vi "Sequence.GetStep.vi"(8 "error in (no error)":errorcluster, 9 "Step #":u16, 10 "Sequence Data":T1[](array[typedef])) -> (0 "error out":errorcluster, 2 "AO [ ]":cluster{"IO Name":string, "IO Value":variant}[](array[cluster]), 3 "DO [ ]":cluster{"IO Name":string, "IO Value":variant}[](array[cluster]))   [LabVIEW 2019]
doc: "Gets a step in the sequence (by it's index in the Sequence Data [ ] array), outputting the AO [] (Analog Outputs) and DO [ ] (Digital Outputs) for that step as separate arrays."
uses:
  typedefs/step.data--Cluster.ctl
  typedefs/step.IO.data--Cluster.ctl
  typedefs/IOType--Enum.ctl
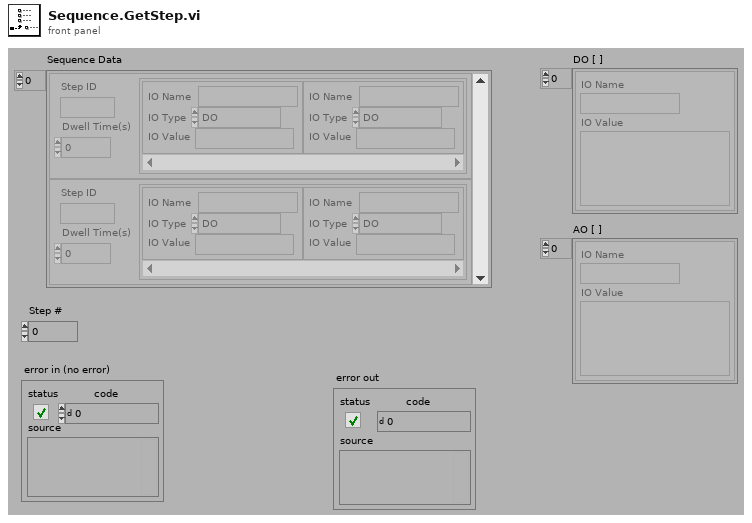
[diagram p1: front panel]
types:
  T1 = typedef "step.data--Cluster.ctl" = cluster{"Step ID":string, "Dwell Time(s)":dbl, "Recipe Step":T2[]}
  T2 = typedef "step.IO.data--Cluster.ctl" = cluster{"IO Name":string, "IO Type":T3, "IO Value":variant}
  T3 = typedef "IOType--Enum.ctl" = enum16{"<Undefined>", "DO", "DI", "AO", "AI"}
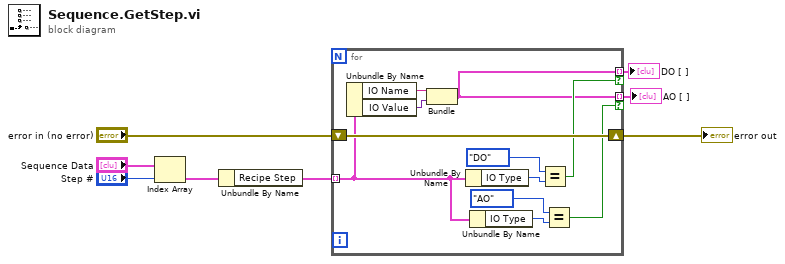
[diagram p0: block diagram]
diagram:
  n1 = Index Array(array="Sequence Data", index="Step #") -> (element=w4:T1)
  n2 = Unbundle By Name(w4) -> ("Recipe Step"=w6:T2[])
  n3 = for {
    tunnel: w6 -> [w10] mode=indexing
    shift-right: [w19] -> w7
    shift-left: "error in (no error)" -> [w19]
    tunnel: [w13] -> w2 mode=indexing if=w16
    tunnel: [w13] -> w1 mode=indexing if=w9
    n4 = Unbundle By Name(w10) -> ("IO Name"=w15:string, "IO Value"=w14:variant)
    n5 = Bundle("IO Name"=w15, "IO Value"=w14) -> (w13:cluster{"IO Name":string, "IO Value":variant})  [unwired: 1 in]
    n6 = Unbundle By Name(w10) -> ("IO Type"=w18:T3)
    n7 = Unbundle By Name(w10) -> ("IO Type"=w11:T3)
    n8 = Equal?(x=enum16{"<Undefined>", "DO", "DI", "AO", "AI"}."DO" ("IO Name"), y=w18) -> (x = y?=w16:bool)
    n9 = Equal?(x=enum16{"<Undefined>", "DO", "DI", "AO", "AI"}."AO" ("IO Name"), y=w11) -> (x = y?=w9:bool)
  }
  "error out" <- w7
  "DO [ ]" <- w2
  "AO [ ]" <- w1
